vi "Pressure to voltage.vi"(0 "Pressure SP":dbl) -> (4 "Voltage":dbl)   [LabVIEW 2019, in "Stand.lvclass"]
uses:
  Stand.lvclass
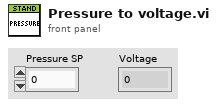
[diagram p1: front panel]
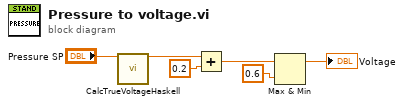
[diagram p0: block diagram]
diagram:
  n1 = call "CalcTrueVoltageHaskell.vi"("Pressure SP"="Pressure SP") -> ("Voltage"=w5:dbl)  [unwired: 14 in]
  n2 = Add(x=w5, y=0.2) -> (x+y=w4:dbl)
  n3 = Max & Min(x=w4, y=0.6) -> (max(x,y)=→"Voltage":dbl)  [unwired: 1 out]
